vi "RT_small3.vi"() -> ()   [LabVIEW 2018]
uses:
  <vilib>/Platform/TimedLoop/XDataNode/timing_clust.ctl
  <vilib>/Platform/TimedLoop/XDataNode/nitl_modes.ctl
  <vilib>/Platform/TimedLoop/XDataNode/wakeup.ctl
  <vilib>/FPGAPlugInAG/myRIO-1900/niLvFpga_Open_myRIO-1900.vi
  <vilib>/rvi/interface/common/dynamic/niFpgaDynamicAddResources.vi
  <vilib>/Utility/error.llb/Error Cluster From Error Code.vi
  <vilib>/rvi/errors/niLvFpgaAdjustHostInterfaceError.vi
  <vilib>/addons/control/pid/pid.llb/PID (DBL).vi
  <vilib>/FPGAPlugInAG/Dynamic/niLvFpga_Close_Dynamic.vi
  <vilib>/platform/TimedLoop/XDataNode/XDataNode.xnode
  <vilib>/rvi/interface/nirviOpenFPGA/nirviOpenFPGA.xnode
  FPGA Bitfiles/DQNcarpolelvsim_FPGATarget_FPGAsmall2_d4itNFSFwjs.lvbitx
  FPGA_small2.vi
  <vilib>/rvi/interface/nirviReadWriteControl/nirviReadWriteControl.xnode
  <vilib>/rvi/interface/nirviCloseFPGA/nirviCloseFPGA.xnode
  <vilib>/rvi/interface/Simulation/niFpgaSimulationCallBeginRW.vi
  <vilib>/addons/control/pid/NI_PID_pid.lvlib
  NiFpgaLv.dll
  <vilib>/Platform/TimedLoop/XDataNode/XDNodeRunTimeDep.lvlib
panel:
  in  "man":bool
  in  "Slide":i16(slide) scale=-500.0..500.0
  out "pos":T1(graph)
  out "dai Chart":cluster{dbl, dbl, "mean":dbl}(graph)={-4.896466674930966, 0.0024543692606169287, "mean"=0.0003067961575771161}
  in  "selctl":bool
  out "set_pt":i16=-282
  in  "scale":dbl=400.0
  out "pid output":u16(graph)
  in  "dx_sim":dbl=0.05000000000000001
  out "gap_pos":i16=305
  out "states":dbl[](array[numeric])=[-305.0, 12.0, -4.896466674930966, 0.0003067961575771161]
  out "busy":bool=TRUE
  out "off_track":bool
  out "output":u16=53
  in  "output range":cluster{"output high":dbl, "output low":dbl}={"output high"=80.0, "output low"=53.0} {"output low" format="%.2f"; "output high" format="%.2f"}
  in  "dt (s)":dbl=0.001 format="%.3f"
  in  "PID gains":T2={"proportional gain (Kc)"=1.0, "integral time (Ti, min)"=0.0, "derivative time (Td, min)"=0.0006000000000000001} {"derivative time (Td, min)" format="%.5f"; "integral time (Ti, min)" format="%.5f"; "proportional gain (Kc)" format="%.4f"}
  out "speed Chart":i16(graph)=12
  out "position":i16=305
  in  "stop":bool
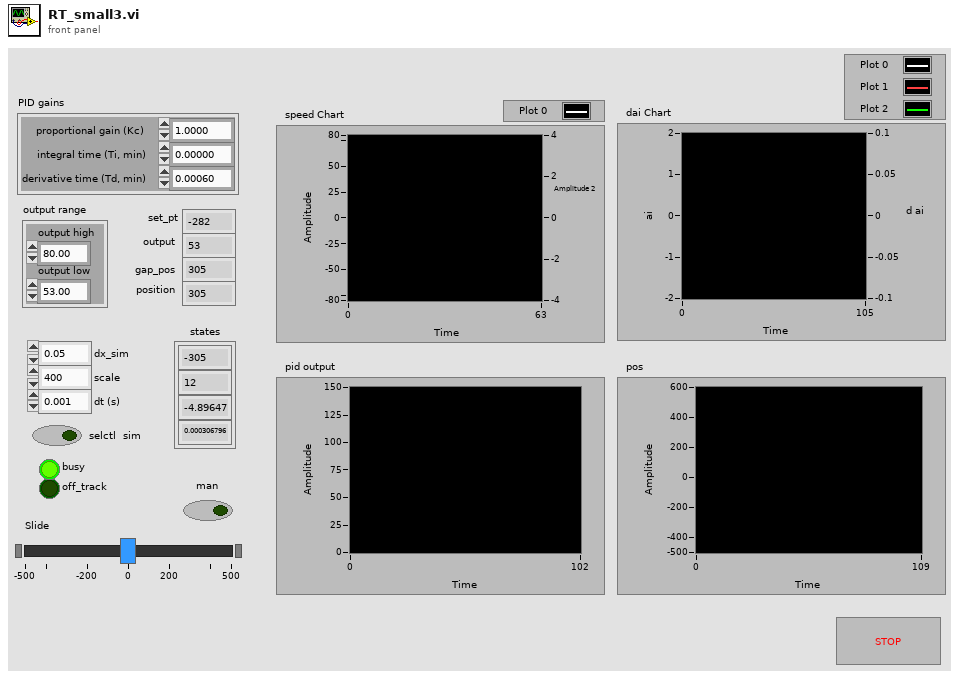
[diagram p1: front panel]
types:
  T1 = cluster{"Slide":i16, "set pt":i16, "position":i16}
  T2 = cluster{"proportional gain (Kc)":dbl, "integral time (Ti, min)":dbl, "derivative time (Td, min)":dbl}
  T3 = typedef "XDNodeRunTimeDep.lvlib/timing_clust.ctl" = cluster{"Expected End [f-1]":u64, "Actual End [f-1]":u64, "Finished Late? [f-1]":bool, "Expected End [i-1]":u64, "Actual End [i-1]":u64, "Finished Late? [i-1]":bool, "Expected Start [i]":u64, "Actual Start [i]":u64, "Expected Start [f]":u64, "Actual Start [f]":u64, "Source Name":string, "Structure Name":string, "Period":i64, "Deadline":i64, "Offset":i64, "Start":i64, "Priority":i32, "Timeout":i32, "Mode":T4, "Wakeup Reason":T5, "Error":errorcluster, "Source Type":string, "Secondary Source Type":string, "Global End Time":u64, "Global Start Time":u64, "Frame Duration":u64, "Iteration Duration":u64, "Assigned CPU":i32, "I/O Scan Engine Mode":u32}
  T4 = typedef "XDNodeRunTimeDep.lvlib/nitl_modes.ctl" = enum32{"No Change", "Process missed periods, maintain original phase", "Discard missed periods, maintain original phase", "Process missed periods, ignore original phase", "Discard missed periods, ignore original phase"}
  T5 = typedef "XDNodeRunTimeDep.lvlib/wakeup.ctl" = enum32{"Normal", "Aborted", "Asynchronous wakeup", "Timing source error", "Timed loop error", "Timeout"}
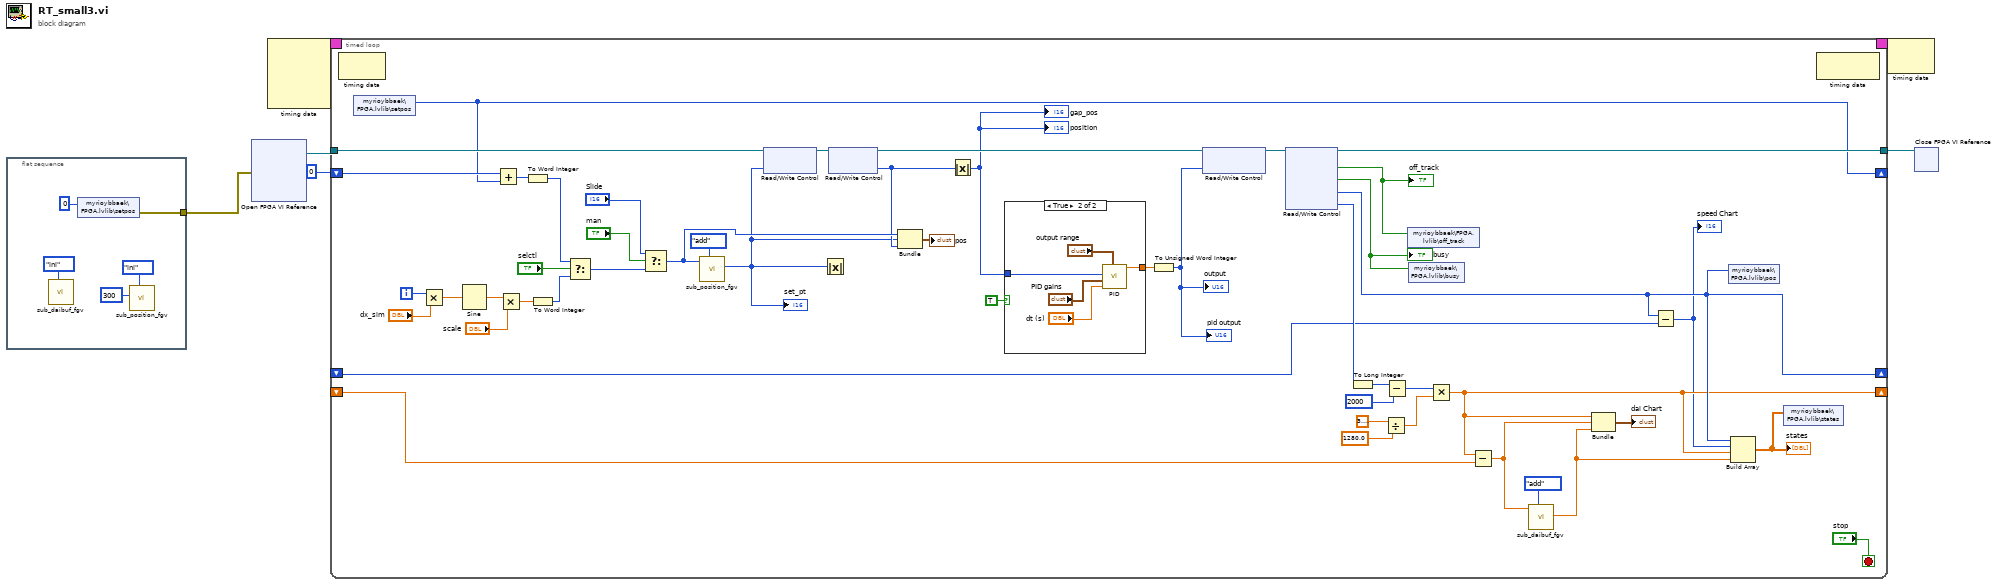
[diagram p0: block diagram]
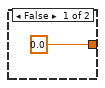
[diagram p2: hidden frame]
diagram:
  n1 = flat-sequence {
    tunnel: [w10] -> w2
    frame #0 {
      n2 = call "sub_daibuf_fgv.vi"("cmd"=enum16{"ini", "add"}."ini") -> ()  [unwired: 9 in, 2 out]
      n3 = shared-variable "myrioybbaek\\FPGA.lvlib\\setpos"(i16 0 ("setpos")) -> (error out=w10:errorcluster)  [unwired: 1 in]
      n4 = call "sub_position_fgv.vi"("cmd"=enum16{"ini", "add"}."ini", "buf size"=300) -> ()  [unwired: 8 in, 2 out]
    }
  }
  n5 = xnode "Open FPGA VI Reference"("error in"=w2) -> ("FPGA VI Reference Out"=w5:refnum<k20>)  [unwired: 1 in, 1 out]
  n6 = node-c288() -> (w4:T3)  [unwired: 4 in]
  n7 = timed-loop {
    tunnel: w5 -> [w60]
    tunnel: [w55] -> w6
    timing: w4 -> [_]
    timing-out: [_] -> w3
    shift-right: [w29] -> _
    shift-left: 0 -> [w30]
    shift-right: [w28] -> _
    shift-left: _ -> [w33]
    shift-right: [w32] -> _
    shift-left: _ -> [w31]
    i -> [w43]
    stop <- "stop" stop-if-true
    n8 = node-c288() -> ()  [unwired: 1 in, 1 out]
    n9 = shared-variable "myrioybbaek\\FPGA.lvlib\\setpos"() -> (w29:i16)  [unwired: 1 in, 1 out]
    n10 = Multiply(x=w43, y="dx_sim") -> (x*y=w41:dbl)
    n11 = Sine(x=w41) -> (sin(x)=w40:dbl)
    n12 = Add(x=w30, y=w29) -> (x+y=w34:i32)
    n13 = Multiply(x=w40, y="scale") -> (x*y=w38:dbl)
    n14 = To Word Integer(number=w34) -> (16bit integer=w35:i16)
    n15 = To Word Integer(number=w38) -> (16bit integer=w36:i16)
    n16 = Select(t=w35, s="selctl", f=w36) -> (s? t:f=w16:i16)
    n17 = Select(t="Slide", s="man", f=w16) -> (s? t:f=w14:i16)
    n18 = call "sub_position_fgv.vi"("cmd"=enum16{"ini", "add"}."add", "data"=w14) -> ("set pt"=w12:i16)  [unwired: 8 in, 1 out]
    "set_pt" <- w12
    n19 = xnode "Read/Write Control"("FPGA VI Reference In"=w60, "set_point"=w12) -> ("FPGA VI Reference Out"=w58:refnum<k20>)  [unwired: 1 in, 1 out]
    n20 = Absolute Value(x=w12) -> ()  [unwired: 1 out]
    n21 = xnode "Read/Write Control"("FPGA VI Reference In"=w58) -> ("FPGA VI Reference Out"=w57:refnum<k20>, "position"=w13:i16)  [unwired: 1 in, 1 out]
    n22 = Bundle("Slide"=w14, "set pt"=w12, "position"=w13) -> (→"pos":T1)  [unwired: 1 in]
    n23 = Absolute Value(x=w13) -> (abs(x)=w23:i16)
    "position" <- w23
    "gap_pos" <- w23
    n24 = case shown="True" TRUE {
      tunnel: [0.0 ("output") w63] -> w37
      tunnel: w23 -> [_ w62]
      frame False {
      }
      frame True {
        n25 = call-poly <vilib>:"PID.vi"("output range"="output range", "dt (s)"="dt (s)", "PID gains"="PID gains", "process variable"=w62) -> ("output"=w63:dbl)  [unwired: 6 in, 1 out]
      }
    }
    n26 = To Unsigned Word Integer(number=w37) -> (unsigned 16bit integer=w19:u16)
    "output" <- w19
    "pid output" <- w19
    n27 = xnode "Read/Write Control"("FPGA VI Reference In"=w57, "dt_pwm_us"=w19) -> ("FPGA VI Reference Out"=w56:refnum<k20>)  [unwired: 1 in, 1 out]
    n28 = xnode "Read/Write Control"("FPGA VI Reference In"=w56) -> ("FPGA VI Reference Out"=w55:refnum<k20>, "off_track"=w53:bool, "busy"=w45:bool, "position"=w32:i16, "AI0"=w44:u16)  [unwired: 1 in, 1 out]
    "off_track" <- w53
    "busy" <- w45
    n29 = To Long Integer(number=w44) -> (32bit integer=w52:i32)
    n30 = Divide(x=3.141592653589793, y=1280.0) -> (x/y=w51:dbl)
    n31 = Subtract(x=w52, y=u16 2000) -> (x-y=w50:i32)
    n32 = shared-variable "myrioybbaek\\FPGA.lvlib\\off_track"(w53) -> ()  [unwired: 1 in, 1 out]
    n33 = shared-variable "myrioybbaek\\FPGA.lvlib\\busy"(w45) -> ()  [unwired: 1 in, 1 out]
    n34 = Multiply(x=w50, y=w51) -> (x*y=w28:dbl)
    n35 = Subtract(x=w28, y=w33) -> (x-y=w25:dbl)
    n36 = call "sub_daibuf_fgv.vi"("cmd"=enum16{"ini", "add"}."add", "data"=w25) -> ("mean"=w18:dbl)  [unwired: 8 in, 1 out]
    n37 = Bundle(w28, w25, "mean"=w18) -> (→"dai Chart":cluster{dbl, dbl, "mean":dbl})  [unwired: 1 in]
    n38 = Subtract(x=w32, y=w31) -> (x-y=w24:i16)
    "speed Chart" <- w24
    n39 = shared-variable "myrioybbaek\\FPGA.lvlib\\pos"(w32) -> ()  [unwired: 1 in, 1 out]
    n40 = Build Array(w32, w24, w28, w18) -> (w46:dbl[])
    "states" <- w46
    n41 = shared-variable "myrioybbaek\\FPGA.lvlib\\states"(w46) -> ()  [unwired: 1 in, 1 out]
    n42 = node-c288() -> ()  [unwired: 1 in, 1 out]
  }
  n43 = node-c288(w3) -> ()  [unwired: 1 out]
  n44 = xnode "Close FPGA VI Reference"("FPGA VI Reference In"=w6) -> ()  [unwired: 1 in, 1 out]
